vi "Check Limit Switch.vi"(8 "Input":dbl, 10 "Bottom LS RefNum Name":string, 11 "Forwards LS RefNum Name":string) -> (3 "Checked Output":dbl)   [LabVIEW 2014]
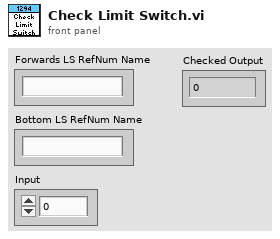
[diagram p1: front panel]
types:
  T1 = typedef "WPI_SwitchDevRef.ctl" = cluster{"DevStatus":errorcluster, "DIO Channel":T2, "Controller":T3, "CntIndex":T4, "Normally Closed":bool}
  T2 = typedef "FPGA_DIOChannel.ctl" = enum8{"DIO 0", "DIO 1", "DIO 2", "DIO 3", "DIO 4", "DIO 5", "DIO 6", "DIO 7", "DIO 8", "DIO 9", "DIO MXP 0", "DIO MXP 1", "DIO MXP 2", "DIO MXP 3", "DIO MXP 4", "DIO MXP 5", "DIO MXP 6", "DIO MXP 7", "DIO MXP 8", "DIO MXP 9", "DIO MXP 10", "DIO MXP 11", "DIO MXP 12", "DIO MXP 13", "DIO MXP 14", "DIO MXP 15", "Invalid"}
  T3 = typedef "FPGA_TypedefDigitalModule.ctl" = enum16{"Controller 1"}
  T4 = typedef "FPGA_CounterCtrSystemIndex.ctl" = enum8{"Ctr 0", "Ctr 1", "Ctr 2", "Ctr 3", "Ctr 4", "Ctr 5", "Ctr 6", "Ctr 7", "Invalid"}
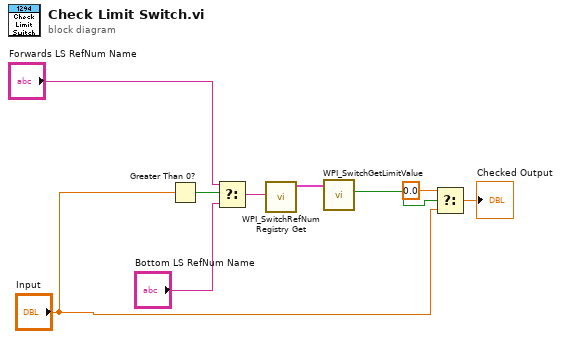
[diagram p0: block diagram]
diagram:
  n1 = Greater Than 0?(x="Input") -> (x > 0?=w9:bool)
  n2 = Select(t="Forwards LS RefNum Name", s=w9, f="Bottom LS RefNum Name") -> (s? t:f=w6:string)
  n3 = call <vilib>:"WPI_SwitchRefNum Registry Get.vi"("refnum name"=w6) -> ("SwitchDevRef"=w5:T1)  [unwired: 9 in, 1 out]
  n4 = call <vilib>:"WPI_SwitchGetLimitValue.vi"("SwitchDevRef"=w5) -> ("Switch Pressed"=w1:bool)  [unwired: 8 in, 2 out]
  n5 = Select(t=0.0, s=w1, f="Input") -> (s? t:f=→"Checked Output":dbl)
